vi "Lab 3 - Monty Hall - Copy.vi"() -> ()   [LabVIEW 2025]
panel:
  in  "Door 3":bool
  in  "Door 2":bool
  in  "Door 1":bool
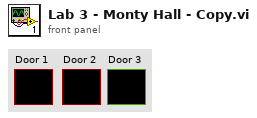
[diagram p1: front panel]
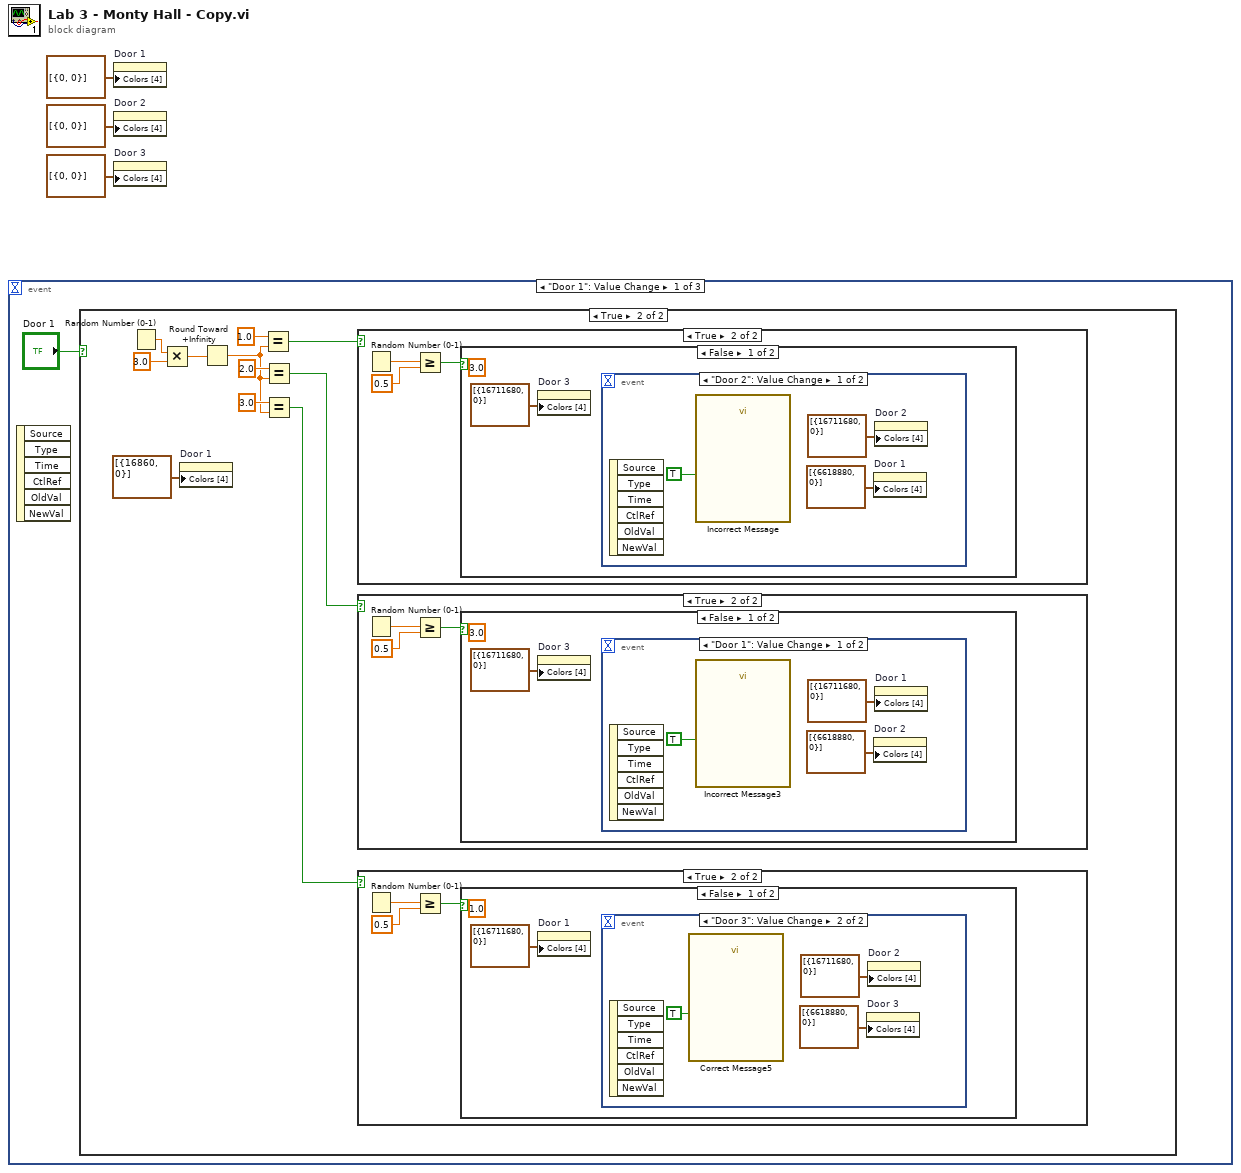
[diagram p0: block diagram]
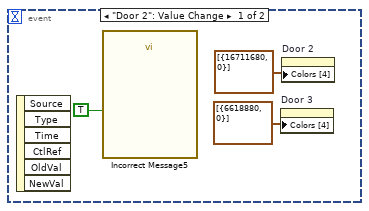
[diagram p4: hidden frame]
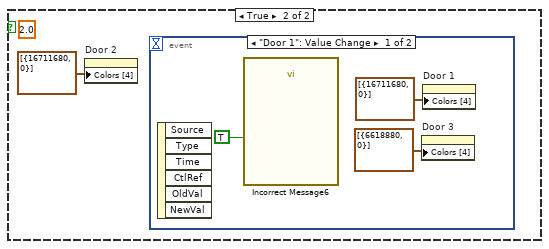
[diagram p5: hidden frame]
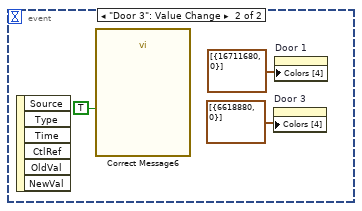
[diagram p6: hidden frame]
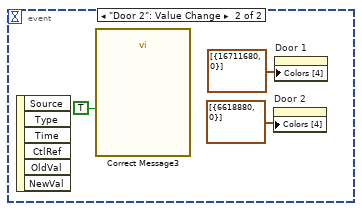
[diagram p8: hidden frame]
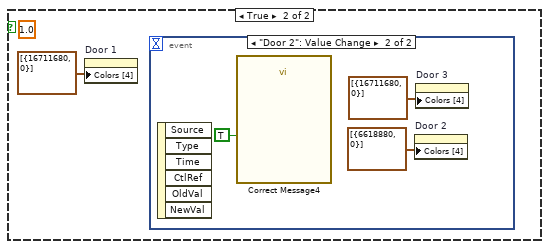
[diagram p9: hidden frame]
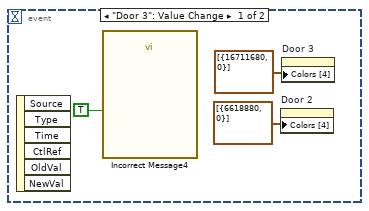
[diagram p10: hidden frame]
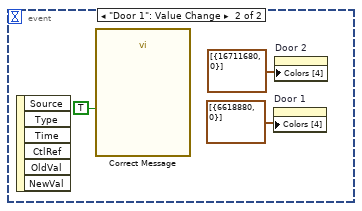
[diagram p12: hidden frame]
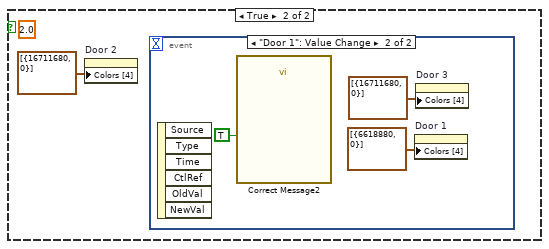
[diagram p13: hidden frame]
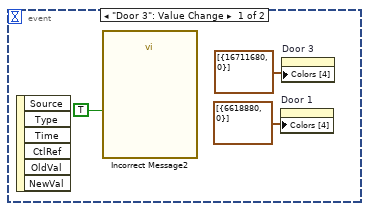
[diagram p14: hidden frame]
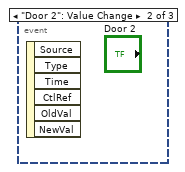
[diagram p15: hidden frame]
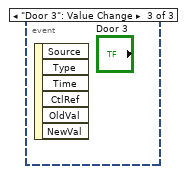
[diagram p16: hidden frame]
diagram:
  n1 = event shown="[0] \"Door 1\": Value Change" {
    selector: _ -> [_ _ _]
    dyn-events: _ -> [_ _ _]
    timeout: _ -> [_ _ _]
    event "Door 1": Value Change {
      n2 = event-data() -> ()  [unwired: 1 in, 6 out]
      n3 = case shown="True" "Door 1" {
        frame False {
        }
        frame True {
          n4 = Random Number (0-1)() -> (number: 0 to 1=w15:dbl)
          n5 = Multiply(x=w15, y=3.0) -> (x*y=w14:dbl)
          n6 = property on="Door 1" class="Bool"("Colors [4]"=cluster{u32, u32}[] [{16860, 0}]) -> ()  [unwired: 2 in, 2 out]
          n7 = Round Toward +Infinity(x=w14) -> (ceil(x): smallest int >= x=w9:dbl)
          n8 = Equal?(x=1.0, y=w9) -> (x = y?=w8:bool)
          n9 = Equal?(x=2.0, y=w9) -> (x = y?=w6:bool)
          n10 = Equal?(x=3.0, y=w9) -> (x = y?=w5:bool)
          n11 = case shown="True" w8 {
            frame False {
            }
            frame True {
              n12 = Random Number (0-1)() -> (number: 0 to 1=w52:dbl)
              n13 = Greater Or Equal?(x=w52, y=0.5) -> (x >= y?=w50:bool)
              n14 = case shown="False" w50 {
                frame False {
                  (unwired) 3.0
                  n15 = property on="Door 3" class="Bool"("Colors [4]"=cluster{u32, u32}[] [{16711680, 0}]) -> ()  [unwired: 2 in, 2 out]
                  n16 = event shown="[0] \"Door 2\": Value Change" {
                    selector: _ -> [_ _]
                    dyn-events: _ -> [_ _]
                    timeout: _ -> [_ _]
                    event "Door 2": Value Change {
                      n17 = event-data() -> ()  [unwired: 1 in, 6 out]
                      n18 = call "Incorrect Message"("Enable"=TRUE) -> ()  [unwired: 9 in, 2 out]
                      n19 = property on="Door 1" class="Bool"("Colors [4]"=cluster{u32, u32}[] [{6618880, 0}]) -> ()  [unwired: 2 in, 2 out]
                      n20 = property on="Door 2" class="Bool"("Colors [4]"=cluster{u32, u32}[] [{16711680, 0}]) -> ()  [unwired: 2 in, 2 out]
                    }
                    event "Door 1": Value Change {
                      n21 = event-data() -> ()  [unwired: 1 in, 6 out]
                      n22 = call "Correct Message"("Enable"=TRUE) -> ()  [unwired: 9 in, 2 out]
                      n23 = property on="Door 1" class="Bool"("Colors [4]"=cluster{u32, u32}[] [{6618880, 0}]) -> ()  [unwired: 2 in, 2 out]
                      n24 = property on="Door 2" class="Bool"("Colors [4]"=cluster{u32, u32}[] [{16711680, 0}]) -> ()  [unwired: 2 in, 2 out]
                    }
                  }
                }
                frame True {
                  (unwired) 2.0
                  n25 = property on="Door 2" class="Bool"("Colors [4]"=cluster{u32, u32}[] [{16711680, 0}]) -> ()  [unwired: 2 in, 2 out]
                  n26 = event shown="[1] \"Door 1\": Value Change" {
                    selector: _ -> [_ _]
                    dyn-events: _ -> [_ _]
                    timeout: _ -> [_ _]
                    event "Door 3": Value Change {
                      n27 = event-data() -> ()  [unwired: 1 in, 6 out]
                      n28 = call "Incorrect Message2"("Enable"=TRUE) -> ()  [unwired: 9 in, 2 out]
                      n29 = property on="Door 1" class="Bool"("Colors [4]"=cluster{u32, u32}[] [{6618880, 0}]) -> ()  [unwired: 2 in, 2 out]
                      n30 = property on="Door 3" class="Bool"("Colors [4]"=cluster{u32, u32}[] [{16711680, 0}]) -> ()  [unwired: 2 in, 2 out]
                    }
                    event "Door 1": Value Change {
                      n31 = event-data() -> ()  [unwired: 1 in, 6 out]
                      n32 = call "Correct Message2"("Enable"=TRUE) -> ()  [unwired: 9 in, 2 out]
                      n33 = property on="Door 1" class="Bool"("Colors [4]"=cluster{u32, u32}[] [{6618880, 0}]) -> ()  [unwired: 2 in, 2 out]
                      n34 = property on="Door 3" class="Bool"("Colors [4]"=cluster{u32, u32}[] [{16711680, 0}]) -> ()  [unwired: 2 in, 2 out]
                    }
                  }
                }
              }
            }
          }
          n35 = case shown="True" w6 {
            frame False {
            }
            frame True {
              n36 = Random Number (0-1)() -> (number: 0 to 1=w35:dbl)
              n37 = Greater Or Equal?(x=w35, y=0.5) -> (x >= y?=w33:bool)
              n38 = case shown="False" w33 {
                frame False {
                  (unwired) 3.0
                  n39 = property on="Door 3" class="Bool"("Colors [4]"=cluster{u32, u32}[] [{16711680, 0}]) -> ()  [unwired: 2 in, 2 out]
                  n40 = event shown="[0] \"Door 1\": Value Change" {
                    selector: _ -> [_ _]
                    dyn-events: _ -> [_ _]
                    timeout: _ -> [_ _]
                    event "Door 1": Value Change {
                      n41 = event-data() -> ()  [unwired: 1 in, 6 out]
                      n42 = call "Incorrect Message3"("Enable"=TRUE) -> ()  [unwired: 9 in, 2 out]
                      n43 = property on="Door 2" class="Bool"("Colors [4]"=cluster{u32, u32}[] [{6618880, 0}]) -> ()  [unwired: 2 in, 2 out]
                      n44 = property on="Door 1" class="Bool"("Colors [4]"=cluster{u32, u32}[] [{16711680, 0}]) -> ()  [unwired: 2 in, 2 out]
                    }
                    event "Door 2": Value Change {
                      n45 = event-data() -> ()  [unwired: 1 in, 6 out]
                      n46 = call "Correct Message3"("Enable"=TRUE) -> ()  [unwired: 9 in, 2 out]
                      n47 = property on="Door 2" class="Bool"("Colors [4]"=cluster{u32, u32}[] [{6618880, 0}]) -> ()  [unwired: 2 in, 2 out]
                      n48 = property on="Door 1" class="Bool"("Colors [4]"=cluster{u32, u32}[] [{16711680, 0}]) -> ()  [unwired: 2 in, 2 out]
                    }
                  }
                }
                frame True {
                  (unwired) 1.0
                  n49 = property on="Door 1" class="Bool"("Colors [4]"=cluster{u32, u32}[] [{16711680, 0}]) -> ()  [unwired: 2 in, 2 out]
                  n50 = event shown="[1] \"Door 2\": Value Change" {
                    selector: _ -> [_ _]
                    dyn-events: _ -> [_ _]
                    timeout: _ -> [_ _]
                    event "Door 3": Value Change {
                      n51 = event-data() -> ()  [unwired: 1 in, 6 out]
                      n52 = call "Incorrect Message4"("Enable"=TRUE) -> ()  [unwired: 9 in, 2 out]
                      n53 = property on="Door 2" class="Bool"("Colors [4]"=cluster{u32, u32}[] [{6618880, 0}]) -> ()  [unwired: 2 in, 2 out]
                      n54 = property on="Door 3" class="Bool"("Colors [4]"=cluster{u32, u32}[] [{16711680, 0}]) -> ()  [unwired: 2 in, 2 out]
                    }
                    event "Door 2": Value Change {
                      n55 = event-data() -> ()  [unwired: 1 in, 6 out]
                      n56 = call "Correct Message4"("Enable"=TRUE) -> ()  [unwired: 9 in, 2 out]
                      n57 = property on="Door 2" class="Bool"("Colors [4]"=cluster{u32, u32}[] [{6618880, 0}]) -> ()  [unwired: 2 in, 2 out]
                      n58 = property on="Door 3" class="Bool"("Colors [4]"=cluster{u32, u32}[] [{16711680, 0}]) -> ()  [unwired: 2 in, 2 out]
                    }
                  }
                }
              }
            }
          }
          n59 = case shown="True" w5 {
            frame False {
            }
            frame True {
              n60 = Random Number (0-1)() -> (number: 0 to 1=w18:dbl)
              n61 = Greater Or Equal?(x=w18, y=0.5) -> (x >= y?=w16:bool)
              n62 = case shown="False" w16 {
                frame False {
                  (unwired) 1.0
                  n63 = property on="Door 1" class="Bool"("Colors [4]"=cluster{u32, u32}[] [{16711680, 0}]) -> ()  [unwired: 2 in, 2 out]
                  n64 = event shown="[1] \"Door 3\": Value Change" {
                    selector: _ -> [_ _]
                    dyn-events: _ -> [_ _]
                    timeout: _ -> [_ _]
                    event "Door 2": Value Change {
                      n65 = event-data() -> ()  [unwired: 1 in, 6 out]
                      n66 = call "Incorrect Message5"("Enable"=TRUE) -> ()  [unwired: 9 in, 2 out]
                      n67 = property on="Door 3" class="Bool"("Colors [4]"=cluster{u32, u32}[] [{6618880, 0}]) -> ()  [unwired: 2 in, 2 out]
                      n68 = property on="Door 2" class="Bool"("Colors [4]"=cluster{u32, u32}[] [{16711680, 0}]) -> ()  [unwired: 2 in, 2 out]
                    }
                    event "Door 3": Value Change {
                      n69 = event-data() -> ()  [unwired: 1 in, 6 out]
                      n70 = call "Correct Message5"("Enable"=TRUE) -> ()  [unwired: 9 in, 2 out]
                      n71 = property on="Door 3" class="Bool"("Colors [4]"=cluster{u32, u32}[] [{6618880, 0}]) -> ()  [unwired: 2 in, 2 out]
                      n72 = property on="Door 2" class="Bool"("Colors [4]"=cluster{u32, u32}[] [{16711680, 0}]) -> ()  [unwired: 2 in, 2 out]
                    }
                  }
                }
                frame True {
                  (unwired) 2.0
                  n73 = property on="Door 2" class="Bool"("Colors [4]"=cluster{u32, u32}[] [{16711680, 0}]) -> ()  [unwired: 2 in, 2 out]
                  n74 = event shown="[0] \"Door 1\": Value Change" {
                    selector: _ -> [_ _]
                    dyn-events: _ -> [_ _]
                    timeout: _ -> [_ _]
                    event "Door 1": Value Change {
                      n75 = event-data() -> ()  [unwired: 1 in, 6 out]
                      n76 = call "Incorrect Message6"("Enable"=TRUE) -> ()  [unwired: 9 in, 2 out]
                      n77 = property on="Door 3" class="Bool"("Colors [4]"=cluster{u32, u32}[] [{6618880, 0}]) -> ()  [unwired: 2 in, 2 out]
                      n78 = property on="Door 1" class="Bool"("Colors [4]"=cluster{u32, u32}[] [{16711680, 0}]) -> ()  [unwired: 2 in, 2 out]
                    }
                    event "Door 3": Value Change {
                      n79 = event-data() -> ()  [unwired: 1 in, 6 out]
                      n80 = call "Correct Message6"("Enable"=TRUE) -> ()  [unwired: 9 in, 2 out]
                      n81 = property on="Door 3" class="Bool"("Colors [4]"=cluster{u32, u32}[] [{6618880, 0}]) -> ()  [unwired: 2 in, 2 out]
                      n82 = property on="Door 1" class="Bool"("Colors [4]"=cluster{u32, u32}[] [{16711680, 0}]) -> ()  [unwired: 2 in, 2 out]
                    }
                  }
                }
              }
            }
          }
        }
      }
    }
    event "Door 2": Value Change {
      n83 = event-data() -> ()  [unwired: 1 in, 6 out]
    }
    event "Door 3": Value Change {
      n84 = event-data() -> ()  [unwired: 1 in, 6 out]
    }
  }
  n85 = property on="Door 1" class="Bool"("Colors [4]"=cluster{u32, u32}[] [{0, 0}]) -> ()  [unwired: 2 in, 2 out]
  n86 = property on="Door 2" class="Bool"("Colors [4]"=cluster{u32, u32}[] [{0, 0}]) -> ()  [unwired: 2 in, 2 out]
  n87 = property on="Door 3" class="Bool"("Colors [4]"=cluster{u32, u32}[] [{0, 0}]) -> ()  [unwired: 2 in, 2 out]
